vi "SubVI.vi"(8 "Signal Type":dbl, 9 "Time":dbl, 10 "Freq":dbl, 11 "Amplitude":dbl) -> (3 "Signal Gen":dbl)   [LabVIEW 2022 SP3]
uses:
  <vilib>/ptbypt/NI_PtbyPt.lvlib
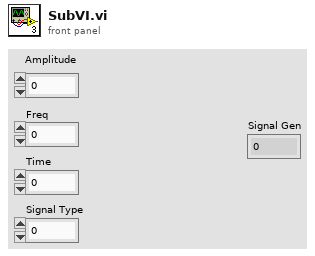
[diagram p1: front panel]
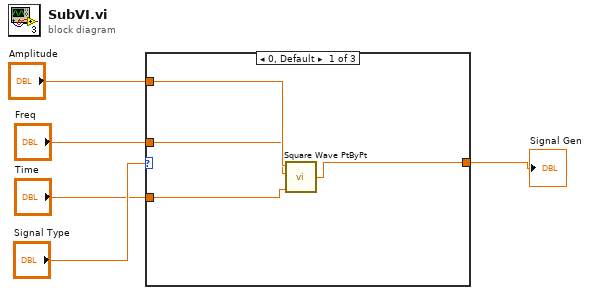
[diagram p0: block diagram]
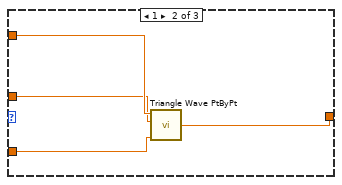
[diagram p2: hidden frame]
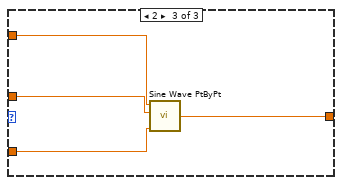
[diagram p3: hidden frame]
diagram:
  n1 = case shown="0, Default" "Signal Type" {
    tunnel: "Amplitude" -> [w9 w13 w17]
    tunnel: "Freq" -> [w8 w12 w16]
    tunnel: "Time" -> [w7 w11 w15]
    tunnel: [w6 w10 w14] -> w1
    frame 0, Default {
      n2 = call <vilib>:"Square Wave PtByPt.vi"("amplitude"=w9, "frequency"=w8, "time"=w7) -> ("square wave"=w6:dbl)  [unwired: 2 in]
    }
    frame 1 {
      n3 = call <vilib>:"Triangle Wave PtByPt.vi"("time"=w11, "frequency"=w12, "amplitude"=w13) -> ("triangle wave"=w10:dbl)  [unwired: 1 in]
    }
    frame 2 {
      n4 = call <vilib>:"Sine Wave PtByPt.vi"("time"=w15, "frequency"=w16, "amplitude"=w17) -> ("sine wave"=w14:dbl)  [unwired: 1 in]
    }
  }
  "Signal Gen" <- w1
